vi "mctl.vi"(7 "LabVIEW Web Service Request":refnum<class "Web Request.lvclass">, 10 "val":u8, 11 "DevID":string) -> ()   [LabVIEW 2014]
doc: "Set a Meerstetter TEC control value. \n\n* 0 = temperature\n* 1 = power"
uses:
  <vilib>/wsapi/Web Request.lvclass
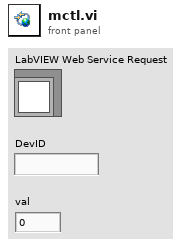
[diagram p1: front panel]
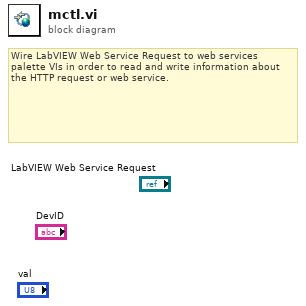
[diagram p0: block diagram]
diagram:
  # "Wire LabVIEW Web Service Request to web services palette VIs in order to read and write information about the HTTP request or web service."
